vi "CoboltLaser_FaultClear.vi"(0 "ComPort":refnum<visa-resource-name>, 3 "CheckResponse":bool=TRUE, 7 "error in (no error)":errorcluster) -> (20 "ComPortOut":refnum<visa-resource-name>, 27 "error out":errorcluster)   [LabVIEW 2012, in "Cobolt.lvclass"]
doc: "Use this template to build a VI to use as a subVI."
uses:
  Template/Cobolt.lvclass
panel:
  out "ResponseOK":bool
  out "Response":string
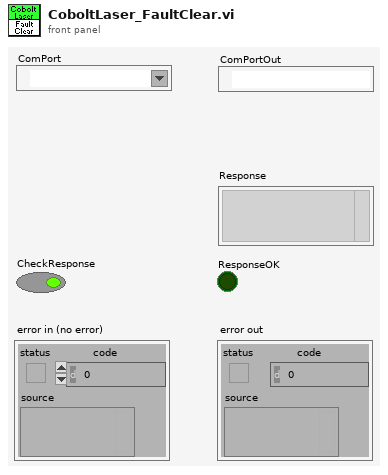
[diagram p1: front panel]
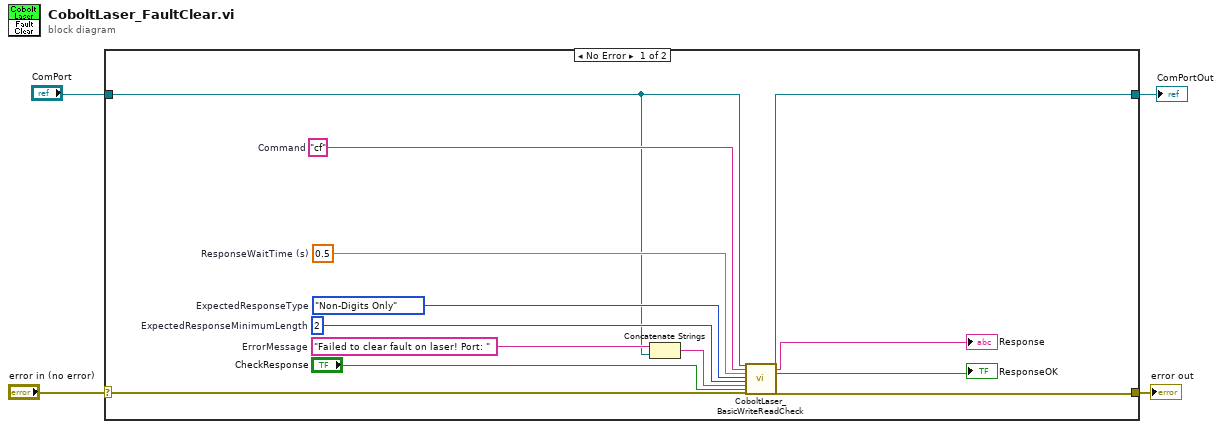
[diagram p0: block diagram]
diagram:
  n1 = case shown="No Error" "error in (no error)" {
    selector: "error in (no error)" -> [w17 w19]
    tunnel: [w16 w19] -> w3
    tunnel: "ComPort" -> [w6 w18]
    tunnel: [w5 w18] -> w1
    frame No Error {
      w13 = 2  # ExpectedResponseMinimumLength
      w14 = enum16{"Any", "Digits Only", "Non-Digits Only"}."Non-Digits Only"  # ExpectedResponseType
      w15 = 0.5  # ResponseWaitTime (s)
      w10 = "Failed to clear fault on laser! Port: "  # ErrorMessage
      w7 = "cf"  # Command
      n2 = Concatenate Strings(w10, w6) -> (w9:string)
      n3 = call "CoboltLaser_BasicWriteReadCheck.vi"("ComPort"=w6, "Command"=w7, "ResponseWaitTime (s)"=w15, "ExpectedResponseType"=w14, "ExpectedResponseMinimumLength"=w13, "ErrorMessage"=w9, "CheckResponse"="CheckResponse", "error in (no error)"=w17) -> ("ComPortOut"=w5:refnum<visa-resource-name>, "Response"=→"Response":string, "ResponseOK"=→"ResponseOK":bool, "error out"=w16:errorcluster)  [unwired: 16 in]
    }
    frame Error {
    }
  }
  "error out" <- w3
  "ComPortOut" <- w1
